vi "TCS_Tx.vi"() -> ()   [LabVIEW 2018]
uses:
  Stream/Stream.lvclass
  RxTx/RxTx.lvclass
panel:
  in  "RxTx in":refnum<class "RxTx.lvclass">
  in  "Stream in":refnum<class "Stream.lvclass">
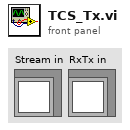
[diagram p1: front panel]
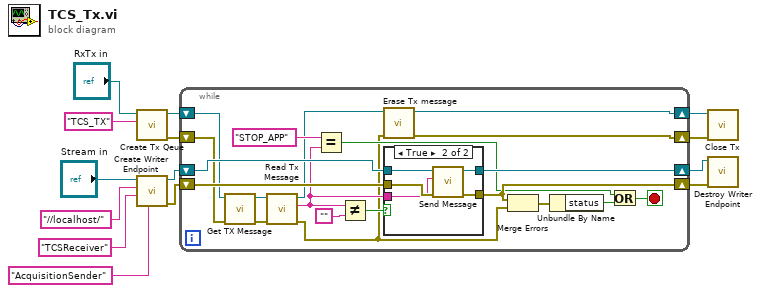
[diagram p0: block diagram]
diagram:
  n1 = call "Create Tx Qeue.vi"("Writer Name"="TCS_TX" ("Reader Name"), "RxTx in"="RxTx in") -> ("error out"=w3:errorcluster, "RxTx out"=w4:refnum<class "RxTx.lvclass">)  [unwired: 8 in]
  n2 = call "Create Writer Endpoint.vi"("writer name"="AcquisitionSender" ("reader name"), "reader name"="TCSReceiver", "IP"="//localhost/" ("Reader Name"), "Stream in"="Stream in") -> ("error out"=w11:errorcluster, "Stream out"=w12:refnum<class "Stream.lvclass">)  [unwired: 6 in]
  n3 = while {
    shift-right: [w30] -> w13
    shift-left: w11 -> [w32]
    shift-right: [w31] -> w14
    shift-left: w12 -> [w33]
    shift-right: [w22] -> w5
    shift-left: w3 -> [w17]
    shift-right: [w23] -> w6
    shift-left: w4 -> [w16]
    stop <- w26 stop-if-true
    n4 = call "Get TX Message.vi"("error in (no error)"=w17, "RxTx in"=w16) -> ("error out"=w18:errorcluster, "RxTx out"=w19:refnum<class "RxTx.lvclass">)  [unwired: 8 in]
    n5 = call "Read Tx Message.vi"("error in (no error)"=w18, "RxTx in"=w19) -> ("error out"=w15:errorcluster, "Tx Message"=w20:string, "RxTx out"=w21:refnum<class "RxTx.lvclass">)  [unwired: 7 in]
    n6 = Equal?(x="STOP_APP", y=w20) -> (x = y?=w28:bool)
    n7 = Not Equal?(x=w20, y="") -> (x != y?=w24:bool)
    n8 = call "Erase Tx message.vi"("error in (no error)"=w15, "RxTx in"=w21) -> ("error out"=w22:errorcluster, "RxTx out"=w23:refnum<class "RxTx.lvclass">)  [unwired: 8 in]
    n9 = case shown="True" w24 {
      tunnel: w33 -> [w36 w38]
      tunnel: w32 -> [w35 w39]
      tunnel: [w36 w41] -> w31
      tunnel: [w35 w40] -> w30
      tunnel: w20 -> [_ w37]
      frame False {
      }
      frame True {
        n10 = call "Send Message.vi"("error in (no error)"=w39, "Message"=w37, "Stream in"=w38) -> ("error out"=w40:errorcluster, "Stream out"=w41:refnum<class "Stream.lvclass">)  [unwired: 7 in]
      }
    }
    n11 = Merge Errors(w30, w15) -> (w34:errorcluster)
    n12 = Unbundle By Name(w34) -> ("status"=w27:bool)
    n13 = Or(x=w28, y=w27) -> (x .or. y?=w26:bool)
  }
  n14 = call "Close Tx.vi"("error in (no error)"=w5, "RxTx in"=w6) -> ()  [unwired: 8 in, 2 out]
  n15 = call "Destroy Writer Endpoint.vi"("error in (no error)"=w13, "Stream in"=w14) -> ()  [unwired: 8 in, 2 out]
